vi "simple read and write test.vi"() -> ()   [LabVIEW 2013]
uses:
  errors/exception.ctl
  errors/context.ctl
  <vilib>/Utility/VariantDataType/GetTypeInfo.vi
  errors/Variant Repository/Write Variant Repository/Write Exception Property.xnode
  errors/exception.lvlib
  <vilib>/Utility/VariantDataType/VariantType.lvlib
  errors/Variant Repository/Read Variant Repository/Read Exception Property.xnode
panel:
  out "exception out":T1 {"code" format="%.0x"}
  out "Replaced? F2":bool
  out "failed t2":bool
  out "failed f2":bool
  out "Replaced t1":bool
  out "Value \"\"":string
  out "failed t":bool
  out "failed  f1":bool
  out "Value sadklm":string
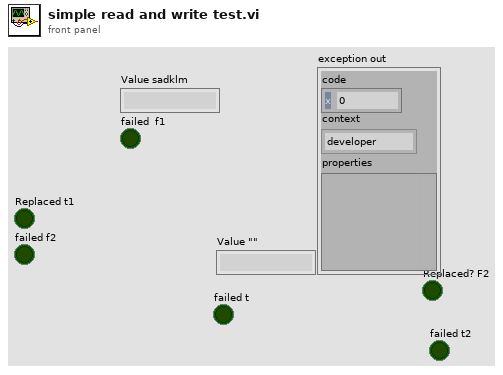
[diagram p1: front panel]
types:
  T1 = typedef "exception.lvlib/exception.ctl" = cluster{"code":i32, "context":T2, "properties":variant}
  T2 = typedef "exception.lvlib/context.ctl" = enum16{"developer", "user interface", "standard", "limited", "deterministic"}
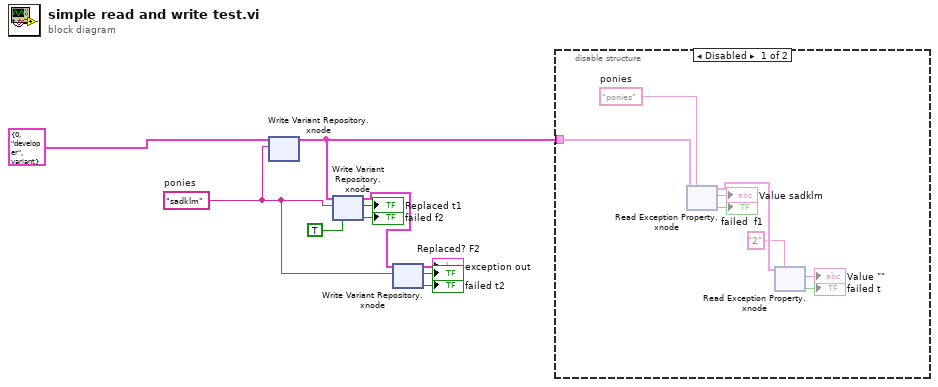
[diagram p0: block diagram]
diagram:
  w2 = "sadklm"  # ponies
  n1 = xnode "Write Variant Repository.xnode"("exception in"=T1 {"code"=0, "context"=enum."developer", "properties"=variant} ("exception"), "Value"=w2) -> ("exception out"=w9:T1)  [unwired: 2 in, 2 out]
  n2 = xnode "Write Variant Repository.xnode"("exception in"=w9, "Value"=w2, "Write Once?"=TRUE) -> ("exception out"=w4:T1, "Replaced?"=→"Replaced t1":bool, "failed"=→"failed f2":bool)  [unwired: 1 in]
  n3 = xnode "Write Variant Repository.xnode"("exception in"=w4, "Value"=w2) -> ("exception out"=→"exception out":T1, "Replaced?"=→"Replaced? F2":bool, "failed"=→"failed t2":bool)  [unwired: 2 in]
  n4 = disable-structure shown="Disabled" {
    disable-tunnel: w9 -> [w11 _]
    frame Disabled {
      w12 = "ponies"  # ponies
      n5 = xnode "Read Exception Property.xnode"("exception in"=w11, "Tag"=w12) -> ("exception out"=w14:T1, "Value"=→"Value sadklm":string, "failed"=→"failed  f1":bool)  [unwired: 1 in]
      n6 = xnode "Read Exception Property.xnode"("exception in"=w14, "Tag"="2") -> ("Value"=→"Value \"\"":string, "failed"=→"failed t":bool)  [unwired: 1 in, 1 out]
    }
    frame Enabled {
    }
  }
